vi "配置读取.vi"(8 "error in (no error)":errorcluster caption="错误输入（无错误）", 11 "Cleaningcycle 输入":refnum<class "Cleaning cycle.lvclass">) -> (0 "error out":errorcluster caption="错误输出", 3 "Cleaningcycle 输出":refnum<class "Cleaning cycle.lvclass">)   [LabVIEW 2022 SP3, in "Cleaning cycle.lvclass"]
uses:
  Cleaning cycle.lvclass
  Cleaning cycle.lvclass/Cleaning cycle.ctl
  <vilib>/Utility/xml.llb/Read From XML File(string).vi
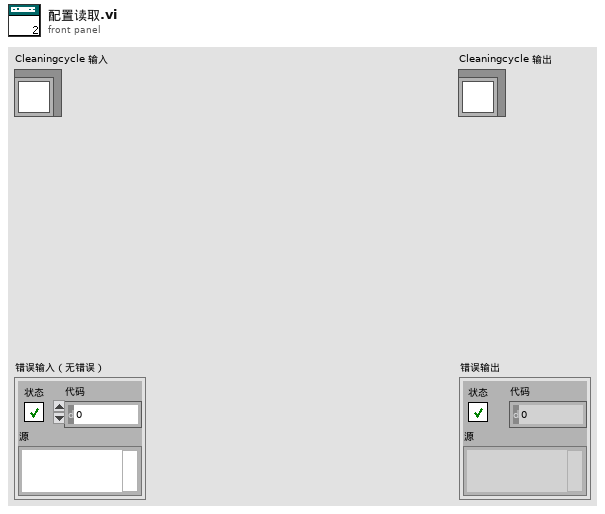
[diagram p1: front panel]
types:
  T1 = typedef "Cleaning cycle.lvclass/State Data.ctl" = cluster{"配置文件路径":path, "简易流程路径":path, "参数列表":cluster{"String":string, "Value":u16}[], "简易流程列表":cluster{"String":string, "Value":u16}[], "配置信息":T2, "命令":cluster{"触发":bool, "周期项":T4}[]}
  T2 = typedef "Cleaning cycle.lvclass/配置信息.ctl" = cluster{"任务列表":T3}
  T3 = typedef "Cleaning cycle.lvclass/任务.ctl" = cluster{"启用":bool, "项":string[][]}
  T4 = typedef "Cleaning cycle.lvclass/周期项.ctl" = cluster{"时":i32, "分":i32, "频次":string, "id":i32, "参数":string, "simpleflowid":i32, "简易流程名称":string}
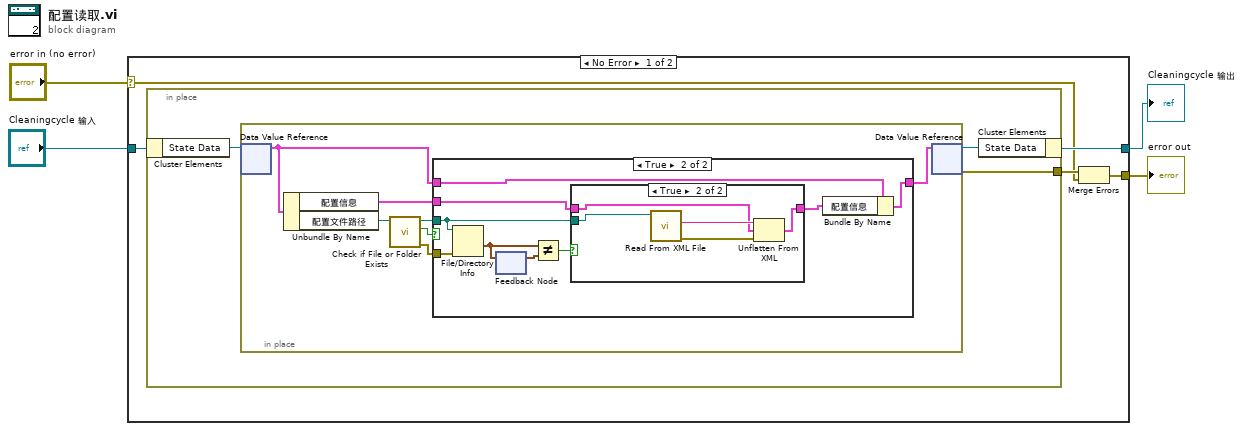
[diagram p0: block diagram]
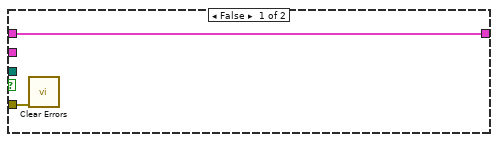
[diagram p2: hidden frame]
diagram:
  n1 = case shown="No Error" "error in (no error)" {
    selector: "error in (no error)" -> [w6 w38]
    tunnel: [w5 w38] -> w3
    tunnel: [w8 w37] -> w1
    tunnel: "Cleaningcycle 输入" -> [w9 w37]
    frame No Error {
      n2 = in-place {
        in-place-border: [w10] -> w7
        n3 = in-place-cluster #1(w9) -> ("State Data"=w12:refnum<data-value>)
        n4 = in-place {
          n5 = in-place-dvr #2(w12) -> (w18:T1)  [unwired: 1 out]
          n6 = Unbundle By Name(w18) -> ("配置信息"=w16:T2, "配置文件路径"=w17:path)
          n7 = call <vilib>:"Check if File or Folder Exists.vi"("path"=w17) -> ("error out"=w13:errorcluster, "file or folder exists?"=w14:bool, "dup path"=w15:path)  [unwired: 8 in]
          n8 = case shown="True" w14 {
            tunnel: [w21 w30] -> w19
            tunnel: w18 -> [w21 w29]
            tunnel: w16 -> [_ w28]
            tunnel: w15 -> [_ w27]
            tunnel: w13 -> [w20 w22]
            frame False {
              n9 = call <vilib>:"Clear Errors.vi"("error in (no error)"=w20) -> ()  [unwired: 5 in, 2 out]
            }
            frame True {
              n10 = File/Directory Info(path=w27, error in=w22) -> (last mod=w24:timestamp)  [unwired: 6 out]
              n11 = feedback-in #3(w24) -> ()
              n12 = feedback #3() -> (w23:timestamp)  [unwired: 1 in]
              n13 = Not Equal?(x=w24, y=w23) -> (x != y?=w26:bool)
              n14 = case shown="True" w26 {
                tunnel: [w31 w34] -> w25
                tunnel: w28 -> [w31 w33]
                tunnel: w27 -> [_ w32]
                frame False {
                }
                frame True {
                  n15 = call-poly <vilib>:"Read From XML File.vi"("XML File Path"=w32) -> ("error out"=w36:errorcluster, "XML Elements"=w35:string)  [unwired: 8 in, 1 out]
                  n16 = Unflatten From XML(xml string=w35, type=w33, error in (no error)=w36) -> (value=w34:T2)  [unwired: 1 out]
                }
              }
              n17 = Bundle By Name(cluster=w29, "配置信息"=w25) -> (w30:T1)
            }
          }
          n18 = in-place-dvr #2(w19) -> (w11:refnum<data-value>, w10:errorcluster)
        }
        n19 = in-place-cluster #1("State Data"=w11) -> (w8:refnum<class "Cleaning cycle.lvclass">)
      }
      n20 = Merge Errors(w7, w6) -> (w5:errorcluster)
    }
    frame Error {
    }
  }
  "error out" <- w3
  "Cleaningcycle 输出" <- w1
